vi "Get HS Speed.vi"(7 "speed":sgl, 8 "error in (no error)":errorcluster, 9 "index":i32, 10 "typ":i32, 11 "channel":i32) -> (0 "error out":errorcluster, 3 "function return":u32, 5 "speed out":sgl)   [LabVIEW 2014, in "atmcd32d.lvlib"]
doc: "unsigned int WINAPI GetHSSpeed(int channel, int typ, int index, float * speed);"
uses:
  atmcd32d.lvlib
  atmcd32d.dll
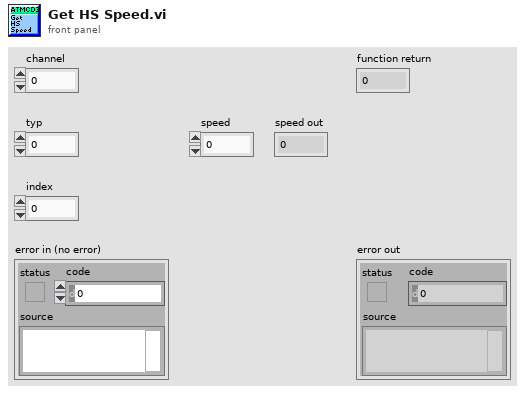
[diagram p1: front panel]
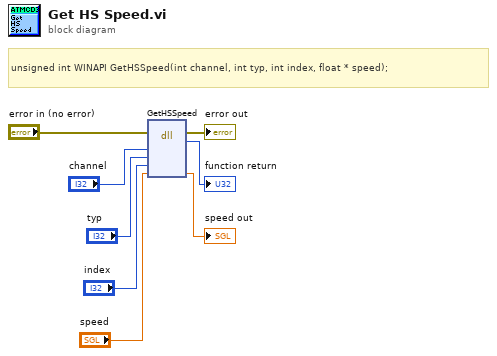
[diagram p0: block diagram]
diagram:
  # "unsigned int WINAPI GetHSSpeed(int channel, int typ, int index, float * speed);"
  n1 = dll-call lib="C:/Users/Bakir/Documents/Lambda2-Testing/lib/Andorlib/atmcd32d.*" fn="GetHSSpeed"(error in="error in (no error)", "channel"="channel", "typ"="typ", "index"="index", "speed"="speed") -> (error out=→"error out":errorcluster, →"function return":u32, "speed"=→"speed out":sgl)  [unwired: 5 in, 1 out]
